vi "MatlabCode.vi"(1 "Writtendatasetname":string, 2 "Datasetname":string) -> (0 "concatenated string":string)   [LabVIEW 2019]
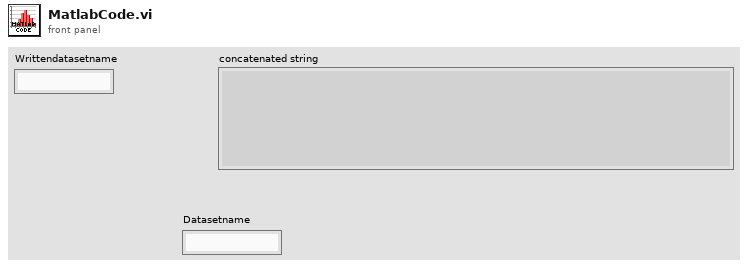
[diagram p1: front panel]
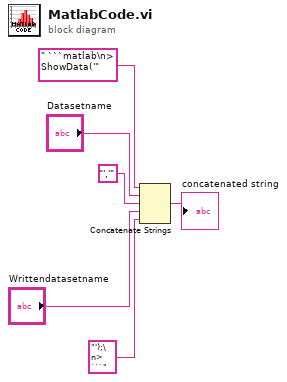
[diagram p0: block diagram]
diagram:
  n1 = Concatenate Strings(" ```matlab\n> ShowData('", "Datasetname", "','" ("string"), "Writtendatasetname", "');\n> ```" ("string")) -> (→"concatenated string":string)
